vi "Get_Instruments_For_Given_Pin.vi"(8 "error in (no error)":errorcluster, 10 "Factory_Data":variant, 11 "Instrument_Factory in":refnum<class "Pin_Instrument_Factory.lvclass">) -> (0 "error out":errorcluster, 2 "Instrument Functions":refnum<class "Function.lvclass">[](array[class]), 3 "Instrument_Factory out":refnum<class "Pin_Instrument_Factory.lvclass">)   [LabVIEW 2020, in "Pin_Instrument_Factory.lvclass"]
uses:
  Pin_Instrument_Factory.lvclass
  Function/Function.lvclass
  Pin_Instrument_Factory.lvclass/Pin_Instrument_Factory.ctl
  <vilib>/MeasurementLink/MeasurementLink Session Management V1/Session Reservation/Session Reservation.lvclass/Session Reservation.ctl
  Instrument/Abstract_Instrument/Abstract_Instrument.lvclass
  <vilib>/MeasurementLink/MeasurementLink Session Management V1/Session Reservation/Get Session Info - NSess .vi
  <vilib>/MeasurementLink/MeasurementLink Session Management V1/Session Reservation/Merge Invalid DVR Error.vi
  <vilib>/MeasurementLink/MeasurementLink Session Management V1/Session Reservation/Is DVR Valid.vi
  <vilib>/MeasurementLink/MeasurementLink Measurement Server/Helpers/Error Strings Global Internal.vi
  <vilib>/Utility/error.llb/Error Cluster From Error Code.vi
  <vilib>/MeasurementLink/MeasurementLink Session Management V1/Session Reservation/Session Reservation.lvclass
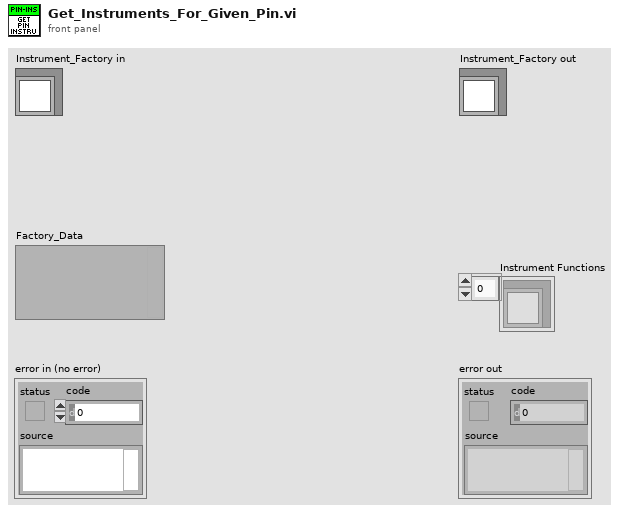
[diagram p1: front panel]
types:
  T1 = typedef "Pin_Instrument_Factory.lvclass/Factory_Data.ctl" = cluster{"Session Reservation":refnum<class "Session Reservation.lvclass">, "Initialize_Info":variant[]}
  T2 = typedef "MeasurementLink Session Management Client.lvlib/ni_measurementlink_sessionmanagement_v1_SessionInformation.ctl" = cluster{"session":T3, "resource_name":string, "channel_list":string, "instrument_type_id":string, "session_exists":bool, "channel_mappings":T4[]}
  T3 = typedef "MeasurementLink Session Management Client.lvlib/nidevice_grpc_Session.ctl" = cluster{"name":string}
  T4 = typedef "MeasurementLink Session Management Client.lvlib/ni_measurementlink_sessionmanagement_v1_ChannelMapping.ctl" = cluster{"pin_or_relay_name":string, "site":i32, "channel":string, "multiplexer_resource_name":string, "multiplexer_route":string}
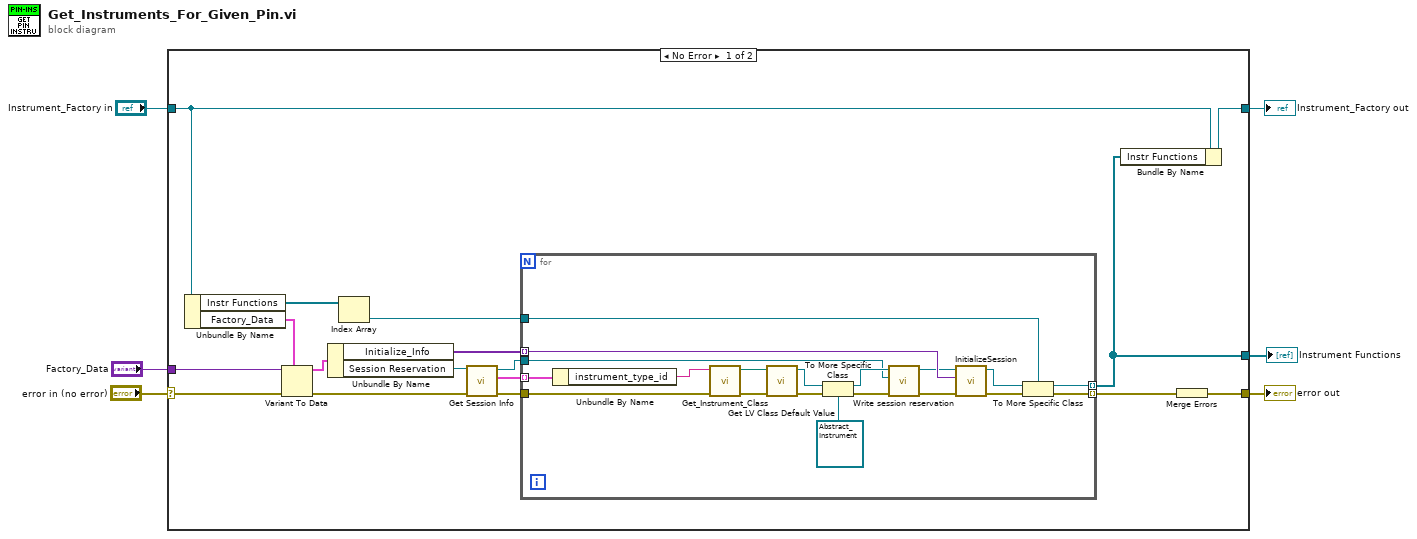
[diagram p0: block diagram]
diagram:
  n1 = case shown="No Error" "error in (no error)" {
    selector: "error in (no error)" -> [w23 w44]
    tunnel: [w13 w44] -> w5
    tunnel: [w10 w43] -> w3
    tunnel: "Instrument_Factory in" -> [w19 w43]
    tunnel: "Factory_Data" -> [w20 _]
    tunnel: [w9 _] -> w1
    frame No Error {
      n2 = Unbundle By Name(w19) -> ("Instr Functions"=w12:refnum<class "Function.lvclass">[], "Factory_Data"=w18:T1)
      n3 = Variant To Data(error in=w23, type=w18, Variant=w20) -> (data=w17:T1, error out=w21:errorcluster)
      n4 = Unbundle By Name(w17) -> ("Initialize_Info"=w8:variant[], "Session Reservation"=w16:refnum<class "Session Reservation.lvclass">)
      n5 = Index Array(array=w12) -> (element=w11:refnum<class "Function.lvclass">)  [unwired: 1 in]
      n6 = call-poly <vilib>:"Get Session Info.vi"("error in"=w21, "session reservation in"=w16) -> ("error out"=w15:errorcluster, "sessions info"=w22:T2[], "session reservation out"=w7:refnum<class "Session Reservation.lvclass">)  [unwired: 7 in]
      n7 = for {
        tunnel: w22 -> [w42] mode=indexing
        tunnel: w15 -> [w37]
        tunnel: [w32] -> w14 mode=indexing
        tunnel: w11 -> [w31]
        tunnel: [w30] -> w9 mode=indexing
        tunnel: w8 -> [w33] mode=indexing
        tunnel: w7 -> [w24]
        n8 = Unbundle By Name(w42) -> ("instrument_type_id"=w39:string)
        n9 = call "Get_Instrument_Class.vi"("error in"=w37, "Instrument_ID"=w39) -> ("error out"=w38:errorcluster, "Instrument class path"=w36:path)  [unwired: 8 in]
        n10 = call <vilib>:"Get LV Class Default Value.vi"("error in (no error)"=w38, "class path"=w36) -> ("error out"=w41:errorcluster, "object"=w40:refnum<class>)  [unwired: 8 in]
        n11 = To More Specific Class(target class=refnum<class "Abstract_Instrument.lvclass"> refnum ("Abstract_Instrument.lvclass"), reference=w40, error in=w41) -> (specific class reference=w26:refnum<class "Abstract_Instrument.lvclass">, error out=w35:errorcluster)
        n12 = call-dynamic "Write session reservation.vi"("error in (no error)"=w35, "Session Reservation.lvclass"=w24, "Abstract_Instrument in"=w26) -> ("error out"=w27:errorcluster, "Abstract_Instrument out"=w25:refnum<class "Abstract_Instrument.lvclass">)  [unwired: 7 in]
        n13 = call-dynamic "InitializeSession.vi"("error in (no error)"=w27, "Initialize_Session"=w33, "Abstract_Instrument in"=w25) -> ("error out"=w28:errorcluster, "Abstract_Instrument out"=w29:refnum<class "Abstract_Instrument.lvclass">)  [unwired: 7 in]
        n14 = To More Specific Class(target class=w31, reference=w29, error in=w28) -> (specific class reference=w30:refnum<class "Function.lvclass">, error out=w32:errorcluster)
      }
      n15 = Bundle By Name(cluster=w19, "Instr Functions"=w9) -> (w10:refnum<class "Pin_Instrument_Factory.lvclass">)
      n16 = Merge Errors(w14) -> (w13:errorcluster)
    }
    frame Error {
    }
  }
  "error out" <- w5
  "Instrument_Factory out" <- w3
  "Instrument Functions" <- w1
